vi "close_port.vi"(8 "error in (no error)":errorcluster, 11 "device_handle":i32) -> (0 "error out":errorcluster, 1 "failstring":string, 2 "closed":bool, 3 "close_response":i32)   [LabVIEW 2014, in "Dali_usb.lvlib"]
uses:
  Dali_usb.lvlib
  dll/DaliBusAccess.dll
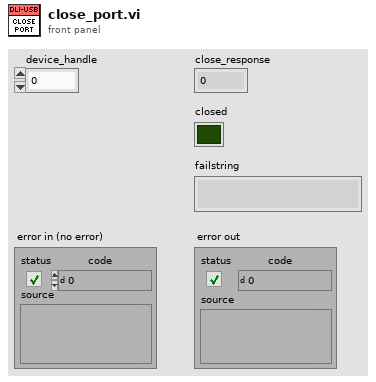
[diagram p1: front panel]
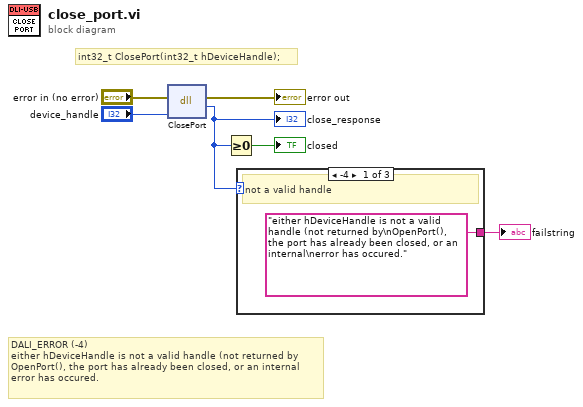
[diagram p0: block diagram]
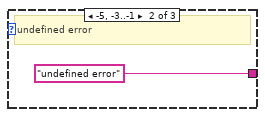
[diagram p2: hidden frame]
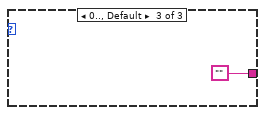
[diagram p3: hidden frame]
diagram:
  # "DALI_ERROR (-4)\neither hDeviceHandle is not a valid handle (not returned by\nOpenPort(), the port has already been closed, or an internal\nerror has occured."
  # "int32_t ClosePort(int32_t hDeviceHandle);"
  n1 = dll-call lib="C:/LTS/app-tde-luminaires/SourceCode/Instruments/Driver_interaction/Dali_usb/Vendor/dll/DaliBusAccess.dll" fn="ClosePort"(error in="error in (no error)", "hDeviceHandle"="device_handle") -> (error out=→"error out":errorcluster, "return type"=w1:i32)  [unwired: 3 in, 1 out]
  "close_response" <- w1
  n2 = Greater Or Equal To 0?(x=w1) -> (x >= 0?=→"closed":bool)
  n3 = case shown="-4" w1 {
    tunnel: ["either hDeviceHandle is not a valid handle (not returned by\nOpenPort(), the port has already been closed, or an internal\nerror has occured." "undefined error" ""] -> w3
    frame -4 {
      # "not a valid handle"
    }
    frame -5, -3..-1 {
      # "undefined error"
    }
    frame 0.., Default {
    }
  }
  "failstring" <- w3
